vi "实验1.vi"() -> ()   [LabVIEW 2021]
uses:
  <vilib>/measure/maspectr.llb/FFT Spectrum (Mag-Phase) for 1 Chan.vi
  <vilib>/measure/maspectr.llb/FFT Spectrum (Mag-Phase) for N Chan.vi
  <vilib>/measure/NI_MABase.lvlib
  <vilib>/measure/NI_MAPro.lvlib
panel:
  out "叠加噪声信号频域":cluster{"f0":dbl, "df":dbl, "magnitude":dbl[]}(graph)
  out "叠加噪声信号时域":waveform(dbl)(graph)
  out "噪声信号频域":cluster{"f0":dbl, "df":dbl, "magnitude":dbl[]}(graph)
  out "噪声信号时域":waveform(dbl)(graph)
  out "解调信号频域":cluster{"f0":dbl, "df":dbl, "magnitude":dbl[]}[](graph)
  out "解调信时域":dynamicdata(graph)
  out "调制信号频域":cluster{"f0":dbl, "df":dbl, "magnitude":dbl[]}(graph)
  out "载波信号频域":cluster{"f0":dbl, "df":dbl, "magnitude":dbl[]}(graph)
  out "基带信号频域":cluster{"f0":dbl, "df":dbl, "magnitude":dbl[]}(graph)
  out "调制信号时域":waveform(dbl)(graph)
  out "基带信号时域":waveform(dbl)(graph)
  out "载波信号时域":waveform(dbl)(graph)
  in  "基带频率":dbl=10.0 format="%0.2p"
  in  "基带幅度":dbl=1.0 caption="基带幅值" format="%0.2p"
  in  "载波频率":dbl=10.0 format="%0.2p"
  in  "载波幅度":dbl=1.0 caption="载波幅值" format="%0.2p"
  in  "采样参数":cluster{"Fs":dbl, "#s":dbl}={"Fs"=1000.0, "#s"=1000.0} caption="采样信息" {"Fs" format="%.2p"}
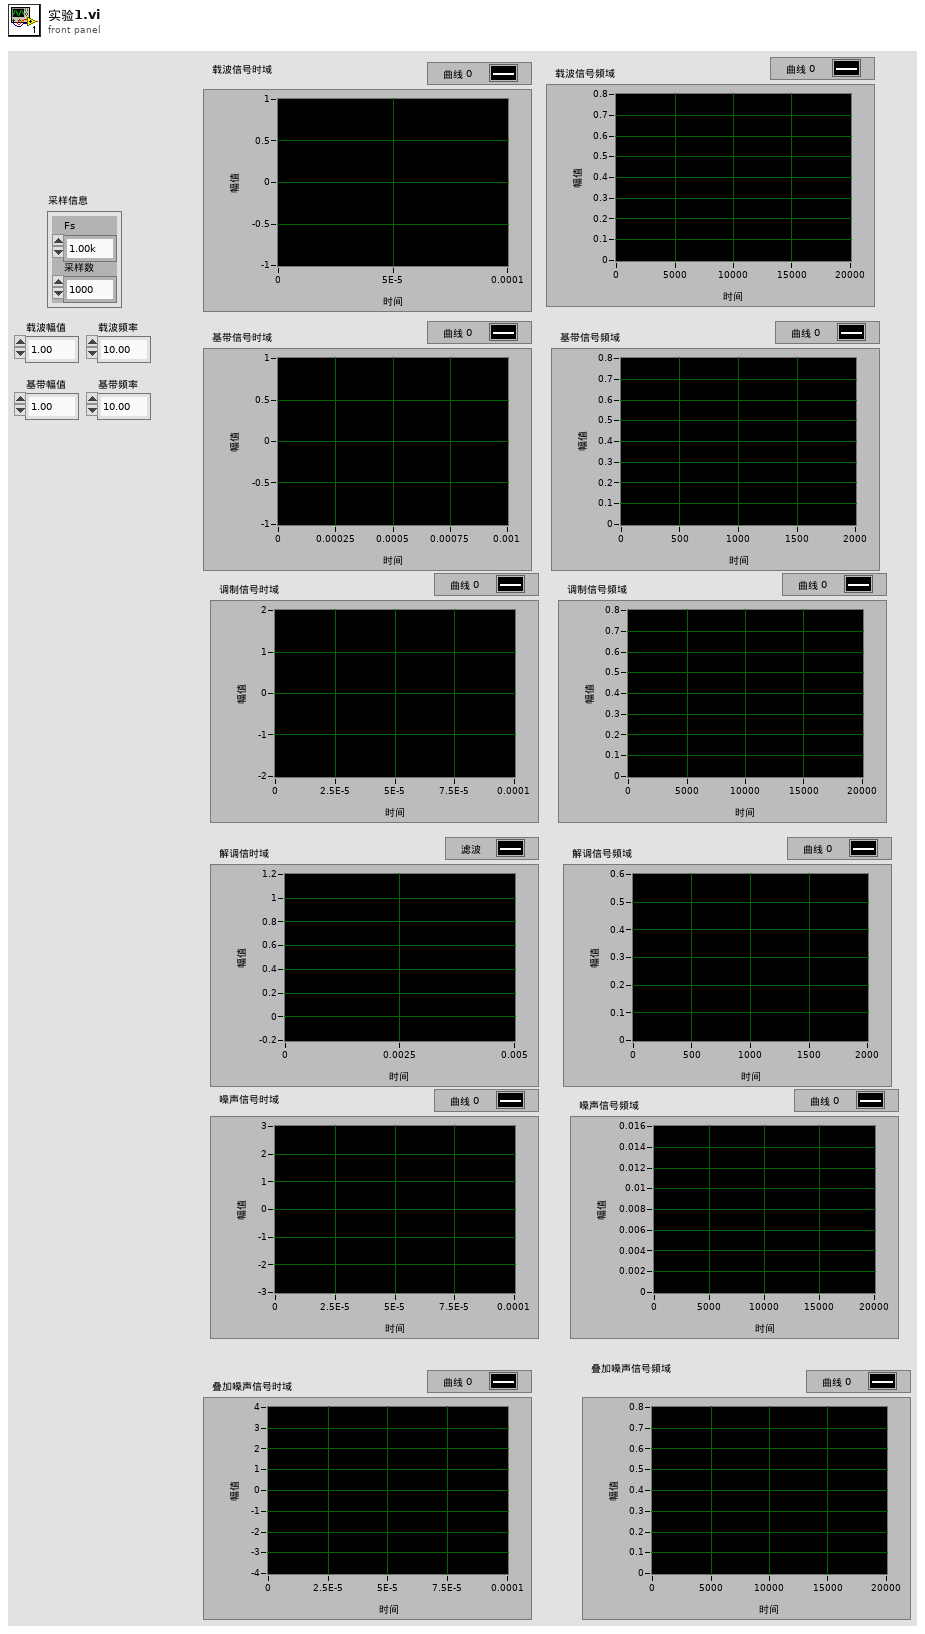
[diagram p1: front panel]
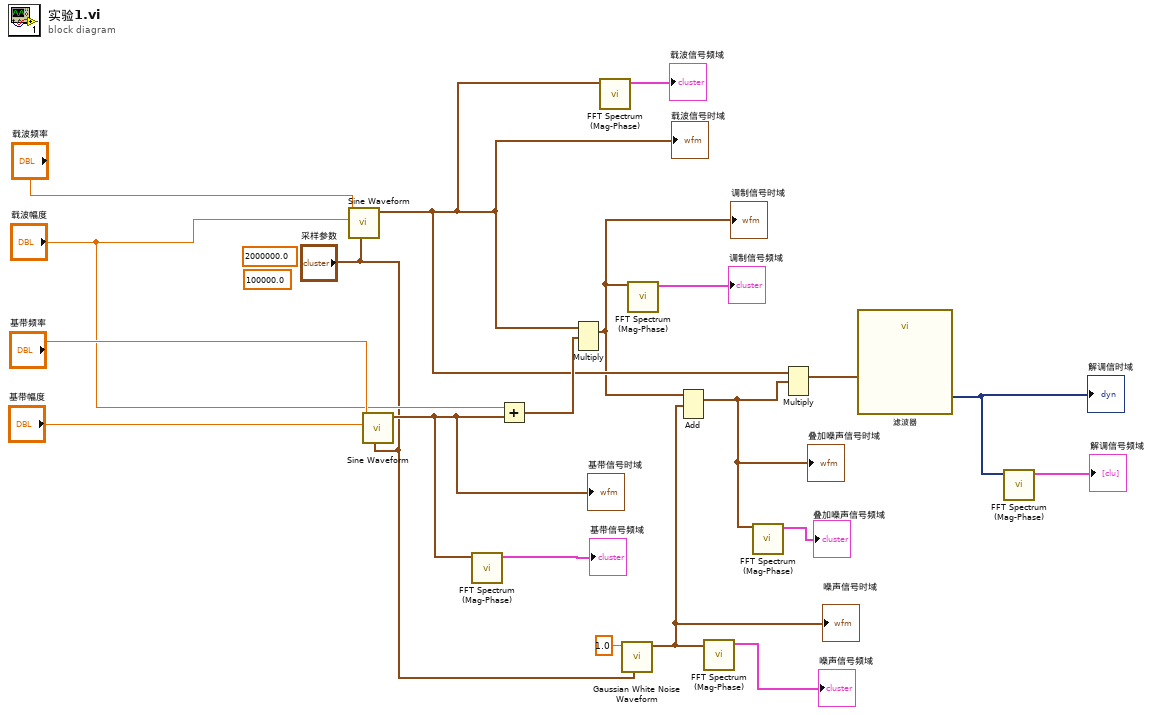
[diagram p0: block diagram]
diagram:
  (unwired) 2000000.0 ("Fs")
  (unwired) 100000.0 ("#s")
  n1 = call <vilib>:"Sine Waveform.vi"("sampling info"="采样参数", "amplitude"="载波幅度", "frequency"="载波频率") -> ("signal out"=w11:waveform(dbl))  [unwired: 7 in, 1 out]
  "载波信号时域" <- w11
  n2 = call <vilib>:"Sine Waveform.vi"("sampling info"="采样参数", "amplitude"="基带幅度", "frequency"="基带频率") -> ("signal out"=w14:waveform(dbl))  [unwired: 7 in, 1 out]
  "基带信号时域" <- w14
  n3 = call-poly <vilib>:"FFT Spectrum (Mag-Phase).vi"("time signal"=w14) -> ("magnitude"=→"基带信号频域":cluster{"f0":dbl, "df":dbl, "magnitude":dbl[]})  [unwired: 6 in, 4 out]
  n4 = Add(x="载波幅度", y=w14) -> (x+y=w16:waveform(dbl))
  n5 = Multiply(1:w16, 2:w11) -> (0:w7:waveform(dbl))  [unwired: 1 in, 1 out]
  "调制信号时域" <- w7
  n6 = call-poly <vilib>:"FFT Spectrum (Mag-Phase).vi"("time signal"=w11) -> ("magnitude"=→"载波信号频域":cluster{"f0":dbl, "df":dbl, "magnitude":dbl[]})  [unwired: 6 in, 4 out]
  n7 = call <vilib>:"Gaussian White Noise Waveform.vi"("sampling info"="采样参数", "standard deviation"=1.0) -> ("signal out"=w4:waveform(dbl))  [unwired: 8 in, 1 out]
  "噪声信号时域" <- w4
  n8 = call-poly <vilib>:"FFT Spectrum (Mag-Phase).vi"("time signal"=w7) -> ("magnitude"=→"调制信号频域":cluster{"f0":dbl, "df":dbl, "magnitude":dbl[]})  [unwired: 6 in, 4 out]
  n9 = Add(1:w4, 2:w7) -> (0:w2:waveform(dbl))  [unwired: 1 in, 1 out]
  "叠加噪声信号时域" <- w2
  n10 = call-poly <vilib>:"FFT Spectrum (Mag-Phase).vi"("time signal"=w4) -> ("magnitude"=→"噪声信号频域":cluster{"f0":dbl, "df":dbl, "magnitude":dbl[]})  [unwired: 6 in, 4 out]
  n11 = call-poly <vilib>:"FFT Spectrum (Mag-Phase).vi"("time signal"=w2) -> ("magnitude"=→"叠加噪声信号频域":cluster{"f0":dbl, "df":dbl, "magnitude":dbl[]})  [unwired: 6 in, 4 out]
  n12 = Multiply(1:w2, 2:w11) -> (0:w10:waveform(dbl))  [unwired: 1 in, 1 out]
  n13 = call "滤波器"("Signal"=w10) -> ("Filtered Signal"=w9:dynamicdata)  [unwired: 9 in, 1 out]
  "解调信时域" <- w9
  n14 = call-poly <vilib>:"FFT Spectrum (Mag-Phase).vi"("time signals"=w9) -> ("magnitudes"=→"解调信号频域":cluster{"f0":dbl, "df":dbl, "magnitude":dbl[]}[])  [unwired: 6 in, 4 out]
